vi "channeldata_digitalwfmpattern.vi"() -> ()   [LabVIEW 2019]
uses:
  <vilib>/Waveform/DWDTOps.llb/Digital Pattern Generator (Ramp).vi
panel:
  out "Digital Waveform Graph":digitalwaveform(graph)={"t0"=timestamp(0 s since 1904-01-01), "dt"=0.001, "Y"={"transitions"=[], "data"=[[0, 0, 0], [0, 0, 1], [0, 1, 0], [0, 1, 1], [1, 0, 0], [1, 0, 1], [1, 1, 0], [1, 1, 1]]}, "error"={"status"=FALSE, "code"=37421928, "source"=""}}
  out "Error Out":errorcluster
  in  "TDMS File":path=path "C:/Python/projects/nitdms/tests/tdms_files/channeldata_digitalwfmpattern.tdms"
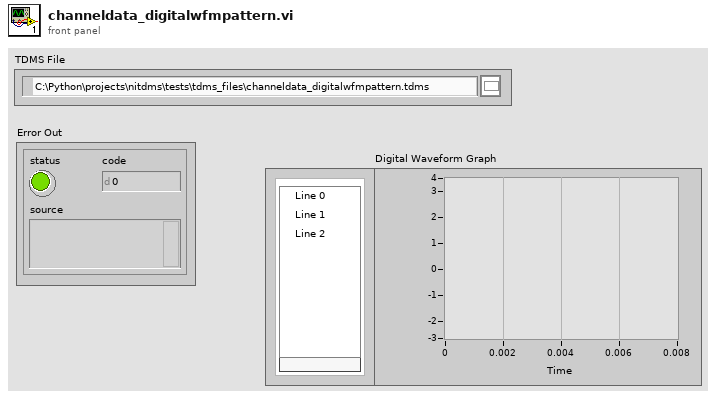
[diagram p1: front panel]
types:
  T1 = enum16{"open", "open or create", "create or replace", "create", "open (read-only)"}
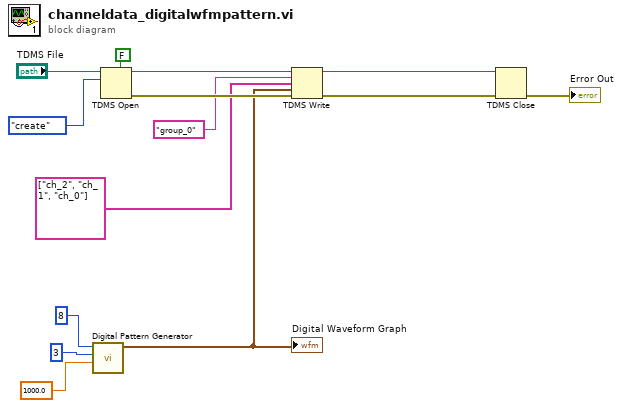
[diagram p0: block diagram]
diagram:
  n1 = call-poly <vilib>:"Digital Pattern Generator.vi"("sample rate"=1000.0, "number of signals"=u32 3, "number of samples"=u32 8) -> ("digital waveform"=w1:digitalwaveform)  [unwired: 7 in, 1 out]
  "Digital Waveform Graph" <- w1
  n2 = TDMS Open(5:FALSE ("create index file? (T)"), 10:T1."create" ("operation (0:open)"), 11:"TDMS File") -> (0:w10:errorcluster, 3:w9:refnum<k34>)  [unwired: 4 in]
  n3 = TDMS Write(0:w9, 5:"group_0", 7:string[] ["ch_2", "ch_1", "ch_0"], 9:w1, 11:w10) -> (4:w7:refnum<k34>, 15:w8:errorcluster)  [unwired: 1 in, 2 out]
  n4 = TDMS Close(8:w8, 11:w7) -> (0:→"Error Out":errorcluster)  [unwired: 1 out]
